vi "stop.vi"(8 "error in (no error)":errorcluster, 11 "Stresing_dual_cam in":refnum<class "Stresing_dual_cam.lvclass">) -> (0 "error out":errorcluster, 3 "Stresing_dual_cam out":refnum<class "Stresing_dual_cam.lvclass">)   [LabVIEW 2019, in "Stresing_dual_cam.lvclass"]
uses:
  Stresing_dual_cam.lvclass
  _cameraBase/_cameraBase.lvclass
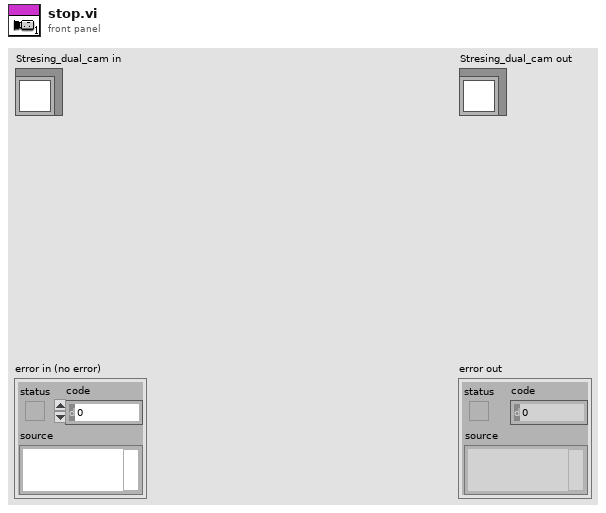
[diagram p1: front panel]
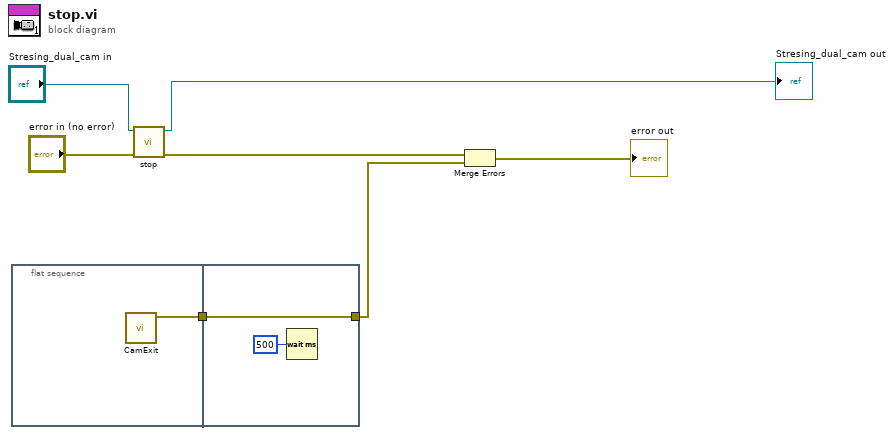
[diagram p0: block diagram]
diagram:
  n1 = flat-sequence {
    tunnel: [w8] -> w3
    tunnel: w3 -> [w9]
    tunnel: [w9] -> w2
    frame #0 {
      n2 = call <instrlib>:"CamExit.vi"() -> ("Camera error out"=w8:errorcluster)  [unwired: 11 in]
    }
    frame #1 {
      n3 = Wait (ms)(milliseconds to wait=u32 500) -> ()  [unwired: 1 out]
    }
  }
  n4 = call-parent "stop.vi"("error in (no error)"="error in (no error)", "_cameraBase in"="Stresing_dual_cam in") -> ("error out"=w4:errorcluster, "_cameraBase out"=→"Stresing_dual_cam out":refnum<class "Stresing_dual_cam.lvclass">)  [unwired: 8 in]
  n5 = Merge Errors(w4, w2) -> (→"error out":errorcluster)
